vi "SetPodOutputVectors.vi"() -> ()   [LabVIEW 2014]
panel:
  in  "Pod Output Vectors":cluster{"Magnitude":dbl, "Direction":dbl}[](array[cluster])
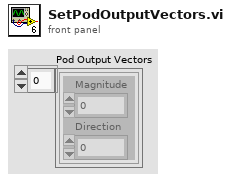
[diagram p1: front panel]
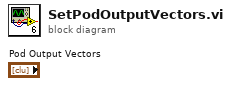
[diagram p0: block diagram]
diagram:
